vi "Image curseur In.vi"(8 "error in (no error)":errorcluster caption="entrée d'erreur (pas d'erreur)", 10 "Image in":u8[][](array[numeric]), 11 "Curseur in":T1) -> (0 "error out":errorcluster caption="sortie d'erreur", 3 "Matrice image":u8[][](array[numeric]))   [LabVIEW 2026]
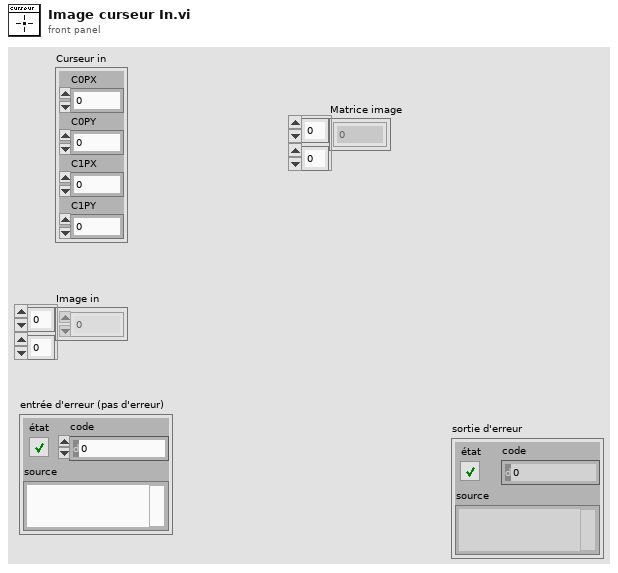
[diagram p1: front panel]
types:
  T1 = cluster{"C0PX":dbl, "C0PY":dbl, "C1PX":dbl, "C1PY":dbl}
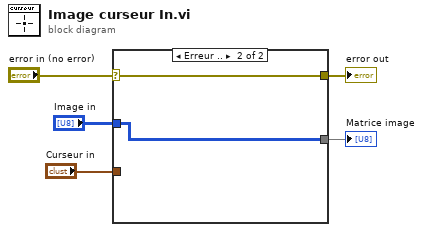
[diagram p0: block diagram]
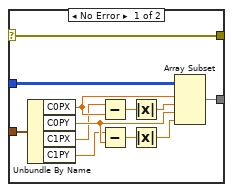
[diagram p2: hidden frame]
diagram:
  n1 = case shown="Erreur .." "error in (no error)" {
    selector: "error in (no error)" -> [w6 w19]
    tunnel: [w17 w18] -> w5
    tunnel: "Image in" -> [w16 w18]
    tunnel: "Curseur in" -> [w7 _]
    tunnel: [w6 w19] -> w1
    frame No Error {
      n2 = Unbundle By Name(w7) -> ("C0PX"=w9:dbl, "C0PY"=w13:dbl, "C1PX"=w8:dbl, "C1PY"=w12:dbl)
      n3 = Subtract(x=w8, y=w9) -> (x-y=w10:dbl)
      n4 = Subtract(x=w12, y=w13) -> (x-y=w14:dbl)
      n5 = Absolute Value(x=w10) -> (abs(x)=w11:dbl)
      n6 = Absolute Value(x=w14) -> (abs(x)=w15:dbl)
      n7 = Array Subset(array=w16, index (row)=w9, length (row)=w11, index (col)=w13, length (col)=w15) -> (w17:u8[][])
    }
    frame Error {
    }
  }
  "Matrice image" <- w5
  "error out" <- w1
